vi "删除特定温度行.vi"(8 "匹配元素":string="20", 10 "数据显示1":string[][](table)) -> (0 "匹配数量":i32, 1 "匹配元素索引":i32[](array[numeric]), 2 "数据显示2":string[][](array[string]))   [LabVIEW 2015]
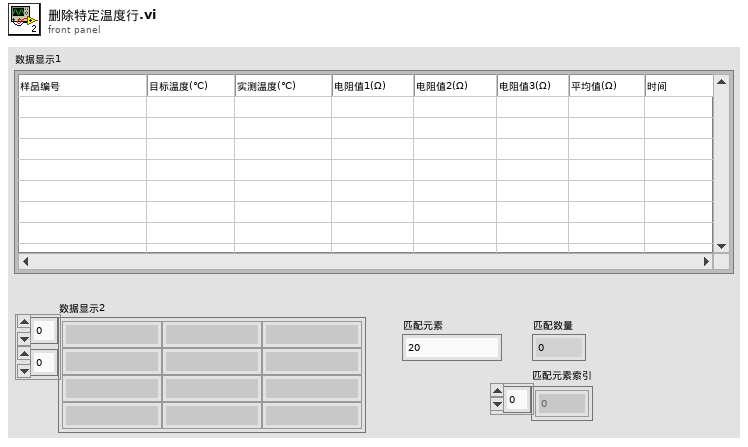
[diagram p1: front panel]
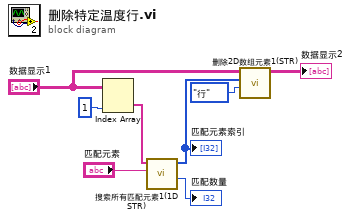
[diagram p0: block diagram]
diagram:
  n1 = Index Array(array="数据显示1", index (col)=1 ("禁用的索引 (列)")) -> (element=w4:string[])  [unwired: 1 in]
  n2 = call "搜索所有匹配元素1(1D STR).vi"("元素"="匹配元素", "数组"=w4) -> ("匹配数量"=→"匹配数量":i32, "匹配元素索引"=w2:i32[])  [unwired: 7 in, 1 out]
  "匹配元素索引" <- w2
  n3 = call "删除2D数组元素1(STR).vi"("选择行列"=enum16{"行", "列"}."行", "索引"=w2, "输入数组"="数据显示1") -> ("剩余元素"=→"数据显示2":string[][])  [unwired: 6 in, 2 out]
